vi "Actor Core.vi"(8 "error in":errorcluster, 11 "Launch IMAQ Display in":refnum<class "Launch File Viewer.lvclass">) -> (0 "error out":errorcluster={"status"=FALSE, "code"=0, "source"="Actor Framework.lvlib:Actor.lvclass:Launch Nested Actor.vi<APPEND>\n\n<b>Complete call chain:</b>\r\n     Actor Framework.lvlib:Actor.lvclass:Launch Nested Actor.vi\r\n     Launch HIJ FileViewer.lvlib:Launch File Viewer.lvclass:Actor Core.vi"}, 3 "Actor out":refnum<class "Actor.lvclass">)   [LabVIEW 2014, in "Launch HIJ FileViewer.lvlib" / "Launch File Viewer.lvclass"]
doc: "(<B>Filename</B>: Actor Framework.lvlib:Actor.lvclass:Actor Core.vi)\n\nReceives messages to the actor, reacts to them, and initiates any error handling that may shut the actor down.\n\nDescendant classes may override this VI to append parallel tasks for the actor to complete while it handles messages. Overrides use the Call Parent Method node."
uses:
  Launch File Viewer.lvclass
  <vilib>/ActorFramework/Actor/Actor.lvclass
  HIJ Vision File Viewer/HIJ Vision File Viewer/HIJ Vision File Viewer.lvclass
  Analyze/Analyze Classes/Analyze Diviation/Analyze BeamDeviation.lvclass
  Analyze/Results and Overlays/Results Beam Deviation/Analyze Results Beam Deviation.lvclass
  Analyze/Analyze Classes/Analyze Distanz/Analyze Distanz.lvclass
  Analyze/Results and Overlays/Results Distance/Analyze Results Distanz.lvclass
  Analyze/Analyze Classes/Analyze Fluence/Analyze Fluence.lvclass
  Analyze/Results and Overlays/Results Fluence/Analyze Results Fluence.lvclass
  Analyze/Analyze Parameter/Analyze Parameter Energy/Analyze Parameter Energy.lvclass
  Analyze/Analyze Parameter/Analyze Parameter Fluence/Analyze Parameter Fluence.lvclass
  Analyze/Results and Overlays/Results Base/Analyze Results Base.lvclass/Analyze Results Base.ctl
  Analyze/Analyze Parameter/Analyze Parameter Energy/Analyze Parameter Energy.lvclass/Analyze Parameter Energy.ctl
  Display Actors/HIJ Vision Display/HIJ Vision Display/HIJ Vision Display.lvclass/HIJ Vision Display.ctl
  Analyze/Results and Overlays/Results Fluence/Analyze Results Fluence.lvclass/Analyze Results Fluence.ctl
  HIJ Vision Application/HIJ Vision Application/HIJ Vision Application.lvclass/HIJ Vision Application.ctl
  <vilib>/ActorFramework/Actor/Actor.lvclass/Actor.ctl
  <vilib>/ActorFramework/Message Enqueuer/Message Enqueuer.lvclass/Message Enqueuer.ctl
  Launch File Viewer Messages/Load Image from File Msg/Load Image from File Msg.lvclass/Load Image from File Msg.ctl
  HIJ Vision Application/HIJ Vision Application Messages/Set Parameter Msg/Set Parameter Msg.lvclass/Set Parameter Msg.ctl
  Analyze/Analyze Parameter/Analyze Parameter Energy/Write Energy.vi
  Analyze/Results and Overlays/Results Base/Write Overlay colors.vi
  Analyze/Results and Overlays/Results Base/Write Overlay_.vi
  Analyze/Results and Overlays/Results Fluence/Write UI Ref Max F.vi
  Display Actors/HIJ Vision Display/HIJ Vision Display/Write Save Report_.vi
  Display Actors/HIJ Vision Display/HIJ Vision Display/Write Show ZoomBtn_.vi
  Display Actors/HIJ Vision Display/HIJ Vision Display/Write WorkDir.vi
  HIJ Vision Application/HIJ Vision Application/Write SubPnl for Display.vi
  HIJ Vision Application/HIJ Vision Application/Write HIJ Vision Display.vi
  HIJ Vision Application/HIJ Vision Application/Write Analyze Objs.vi
  <vilib>/ActorFramework/Message Enqueuer/Init from Existing Queue.vi
  <vilib>/ActorFramework/Message Enqueuer/Enqueue.vi
  Analyze/Analyze Classes/Analyze BaseClass/Analyze BaseClass/Set Result Settings.vi
  Analyze/Analyze Classes/Analyze BaseClass/Analyze BaseClass/Set Parameter.vi
  <vilib>/ActorFramework/Message Priority Queue/Priority Enqueue.vi
  <vilib>/ActorFramework/Message Enqueuer/Message Enqueuer.lvclass
  <vilib>/ActorFramework/Stop Msg/Stop Msg.lvclass
  Launch File Viewer Messages/Load Image from File Msg/Load Image from File Msg.lvclass
  HIJ Vision Application/HIJ Vision Application Messages/Set Parameter Msg/Set Parameter Msg.lvclass
  HIJ Vision Application/HIJ Vision Application/HIJ Vision Application.lvclass
panel:
  in  "Energy":dbl[unit]=10.0
  out "Max F":dbl[unit] format="%#_13g"
  in  "Load Image Report":bool
  in  "Image":path=path "C:/Users/user/Desktop/test/WorkDir"
  in  "Stop Button":bool=TRUE
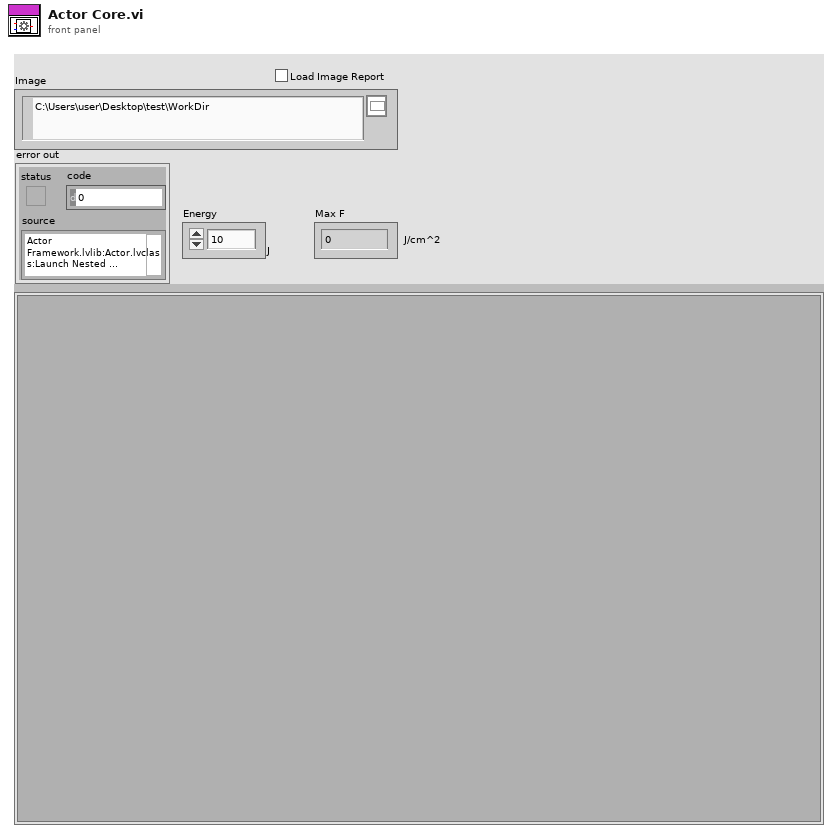
[diagram p1: front panel]
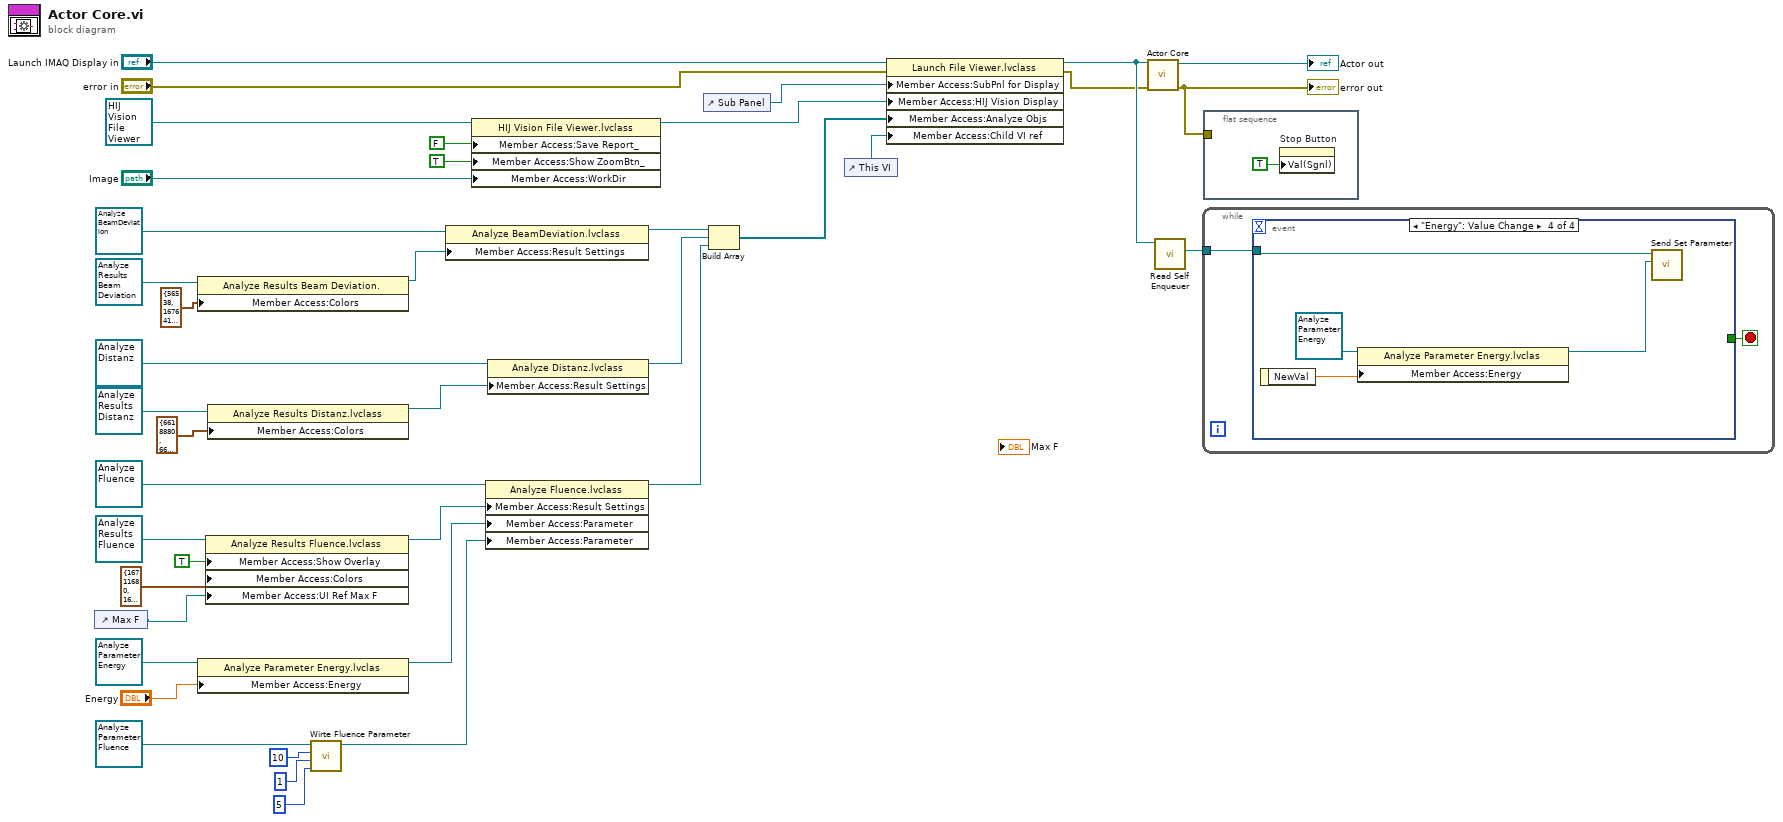
[diagram p0: block diagram]
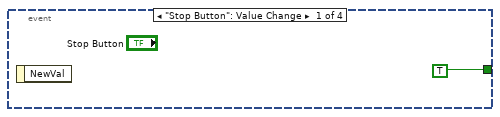
[diagram p2: hidden frame]
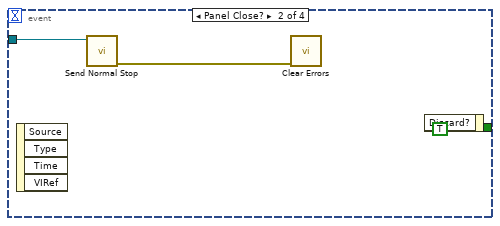
[diagram p3: hidden frame]
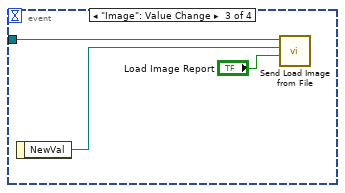
[diagram p4: hidden frame]
diagram:
  n1 = control-ref of="Max F"() -> (w2:refnum<vi>)
  n2 = property class="Analyze Results Beam Deviation."(reference=refnum<class "Analyze Results Beam Deviation.lvclass"> refnum ("Analyze Results Beam Deviation.lvclass"), "Member Access:Colors"=cluster{"Border":u32, "Text":u32} {"Border"=56538, "Text"=16764160} ("Colors")) -> (reference out=w16:refnum<class "Analyze Results Beam Deviation.lvclass">)  [unwired: 1 in, 1 out]
  n3 = property class="Analyze Parameter Energy.lvclas"(reference=refnum<class "Analyze Parameter Energy.lvclass"> refnum ("Analyze Parameter Energy.lvclass"), "Member Access:Energy"="Energy") -> (reference out=w20:refnum<class "Analyze Parameter Energy.lvclass">)  [unwired: 1 in, 1 out]
  n4 = property class="Analyze Results Fluence.lvclass"(reference=refnum<class "Analyze Results Fluence.lvclass"> refnum ("Analyze Results Fluence.lvclass"), "Member Access:Show Overlay"=TRUE ("bOverlay"), "Member Access:Colors"=cluster{"Border":u32, "Text":u32} {"Border"=16711680, "Text"=16448250} ("Colors"), "Member Access:UI Ref Max F"=w2) -> (reference out=w14:refnum<class "Analyze Results Fluence.lvclass">)  [unwired: 1 in, 1 out]
  n5 = property class="Analyze Results Distanz.lvclass"(reference=refnum<class "Analyze Results Distanz.lvclass"> refnum ("Analyze Results Distanz.lvclass"), "Member Access:Colors"=cluster{"Border":u32, "Text":u32} {"Border"=6618880, "Text"=6618880} ("Colors")) -> (reference out=w17:refnum<class "Analyze Results Distanz.lvclass">)  [unwired: 1 in, 1 out]
  n6 = call "Wirte Fluence Parameter.vi"("#of Areas"=5, "#Overlays"=1, "Size of region (px)"=10, "Analyze Parameter Fluence in"=refnum<class "Analyze Parameter Fluence.lvclass"> refnum ("Analyze Parameter Fluence.lvclass")) -> ("Analyze Parameter Fluence out"=w22:refnum<class "Analyze Parameter Fluence.lvclass">)  [unwired: 7 in]
  n7 = property class="Analyze BeamDeviation.lvclass"(reference=refnum<class "Analyze BeamDeviation.lvclass"> refnum ("Analyze.lvlib:Analyze BeamDeviation.lvclass"), "Member Access:Result Settings"=w16) -> (reference out=w15:refnum<class "Analyze BeamDeviation.lvclass">)  [unwired: 1 in, 1 out]
  n8 = property class="HIJ Vision File Viewer.lvclass"(reference=refnum<class "HIJ Vision File Viewer.lvclass"> refnum ("HIJ Vision File Viewer.lvlib:HIJ Vision File Viewer.lvclass"), "Member Access:Save Report_"=FALSE ("Save Report_"), "Member Access:Show ZoomBtn_"=TRUE ("Show ZoomBtn_"), "Member Access:WorkDir"="Image") -> (reference out=w29:refnum<class "HIJ Vision File Viewer.lvclass">)  [unwired: 1 in, 1 out]
  n9 = property class="Analyze Fluence.lvclass"(reference=refnum<class "Analyze Fluence.lvclass"> refnum ("Analyze.lvlib:Analyze Fluence.lvclass"), "Member Access:Result Settings"=w14, "Member Access:Parameter"=w20, "Member Access:Parameter"=w22) -> (reference out=w27:refnum<class "Analyze Fluence.lvclass">)  [unwired: 1 in, 1 out]
  n10 = property class="Analyze Distanz.lvclass"(reference=refnum<class "Analyze Distanz.lvclass"> refnum ("Analyze.lvlib:Analyze Distanz.lvclass"), "Member Access:Result Settings"=w17) -> (reference out=w26:refnum<class "Analyze Distanz.lvclass">)  [unwired: 1 in, 1 out]
  n11 = control-ref of="Sub Panel"() -> (w28:refnum<vi>)
  n12 = Build Array(w15, w26, w27) -> (w3:refnum<class "Analyze BaseClass.lvclass">[])
  n13 = control-ref of="This VI"() -> (w1:refnum<vi>)
  n14 = property class="Launch File Viewer.lvclass"(reference="Launch IMAQ Display in", error in="error in", "Member Access:SubPnl for Display"=w28, "Member Access:HIJ Vision Display"=w29, "Member Access:Analyze Objs"=w3, "Member Access:Child VI ref"=w1) -> (reference out=w32:refnum<class "Launch File Viewer.lvclass">, error out=w30:errorcluster)
  n15 = call-parent "Actor Core.vi"("error in"=w30, "Launch IMAQ Display in"=w32) -> ("error out"=w39:errorcluster, "Actor out"=→"Actor out":refnum<class "Actor.lvclass">)  [unwired: 8 in]
  "error out" <- w39
  n16 = call <vilib>:"Read Self Enqueuer.vi"("Actor"=w32) -> ("Self Enqueuer"=w38:refnum<class "Message Enqueuer.lvclass">)  [unwired: 10 in]
  n17 = while {
    tunnel: w38 -> [w41]
    stop <- w42 stop-if-true
    n18 = event shown="[3] \"Energy\": Value Change" {
      selector: _ -> [_ _ _ _]
      dyn-events: _ -> [_ _ _ _]
      timeout: _ -> [_ _ _ _]
      tunnel: [TRUE TRUE _ _] -> w42
      tunnel: w41 -> [_ w45 w49 w51]
      event "Stop Button": Value Change {
        n19 = event-data() -> ()  [unwired: 1 in, 1 out]
      }
      event Panel Close? {
        n20 = event-data() -> ()  [unwired: 1 in, 4 out]
        n21 = call <vilib>:"Send Normal Stop.vi"("Message Enqueuer"=w45) -> ("error out"=w44:errorcluster)  [unwired: 10 in]
        n22 = call <vilib>:"Clear Errors.vi"("error in (no error)"=w44) -> ()  [unwired: 5 in, 2 out]
        n23 = event-data() -> ()  [unwired: 2 in, 1 out]
      }
      event "Image": Value Change {
        n24 = event-data() -> ("NewVal"=w48:path)  [unwired: 1 in]
        n25 = call "Send Load Image from File.vi"("Load Report"="Load Image Report", "Image"=w48, "Message Enqueuer"=w49) -> ()  [unwired: 7 in, 2 out]
      }
      event "Energy": Value Change {
        n26 = event-data() -> ("NewVal"=w52:dbl[unit])  [unwired: 1 in]
        n27 = property class="Analyze Parameter Energy.lvclas"(reference=refnum<class "Analyze Parameter Energy.lvclass"> refnum ("Analyze Parameter Energy.lvclass"), "Member Access:Energy"=w52) -> (reference out=w50:refnum<class "Analyze Parameter Energy.lvclass">)  [unwired: 1 in, 1 out]
        n28 = call "Send Set Parameter.vi"("Parameter"=w50, "Message Enqueuer"=w51) -> ()  [unwired: 8 in, 2 out]
      }
    }
  }
  n29 = flat-sequence {
    tunnel: w39 -> [_]
    frame #0 {
      n30 = property on="Stop Button" class="Bool (strict)"("Val(Sgnl)"=TRUE) -> ()  [unwired: 2 in, 2 out]
    }
  }
